vi "Test all Data Types in Variant.vi"() -> ()   [LabVIEW 2013]
uses:
  <vilib>/drjdpowell/Messenging/Core Messages/Message/MSG.lvclass
  <vilib>/drjdpowell/Messenging/Core Messages/Message/MSG.lvclass/MSG.ctl
  <vilib>/drjdpowell/Messenging/Core Messages/MSG Library/Write Message (dataless).vi
  <vilib>/drjdpowell/Messenging/Core Messages/MSG Library/Extract (no data).vi
  <vilib>/drjdpowell/Messenging/Core Messages/Message/Label Message.vi
  <vilib>/drjdpowell/Messenging/Core Messages/Message/Overwrite Reply Address.vi
  <vilib>/drjdpowell/Messenging/Core Messengers/Send/Send.lvclass
  JSONtext.lvlib
  <vilib>/drjdpowell/Messenging/Core Messages/MSG Library/SendMSG.lvlib
panel:
  out "x = y?":T1
  out "Occurence valid":bool
  out "error out":errorcluster
  out "Queue refun Valid":bool
  out "<JSON>":string
  out "subVariant":variant
  out "Label":string
  out "Variant out":variant
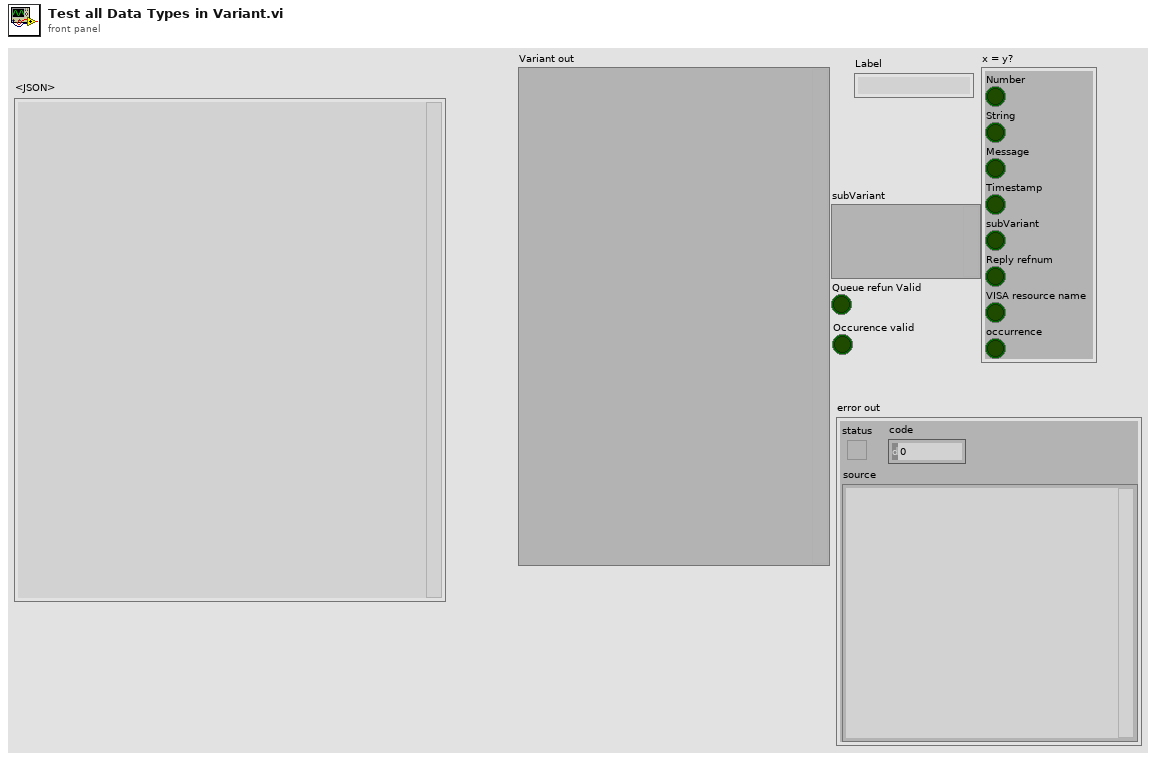
[diagram p1: front panel]
types:
  T1 = cluster{"Number":bool, "String":bool, "Message":bool, "Timestamp":bool, "subVariant":bool, "Reply refnum":bool, "VISA resource name":bool, "occurrence":bool}
  T2 = cluster{"Number":i32, "String":string, "Message":refnum<class "MSG.lvclass">, "Timestamp":timestamp, "subVariant":variant, "Reply refnum":refnum<queue>, "VISA resource name":refnum<visa-resource-name>, "occurrence":refnum<k4>}
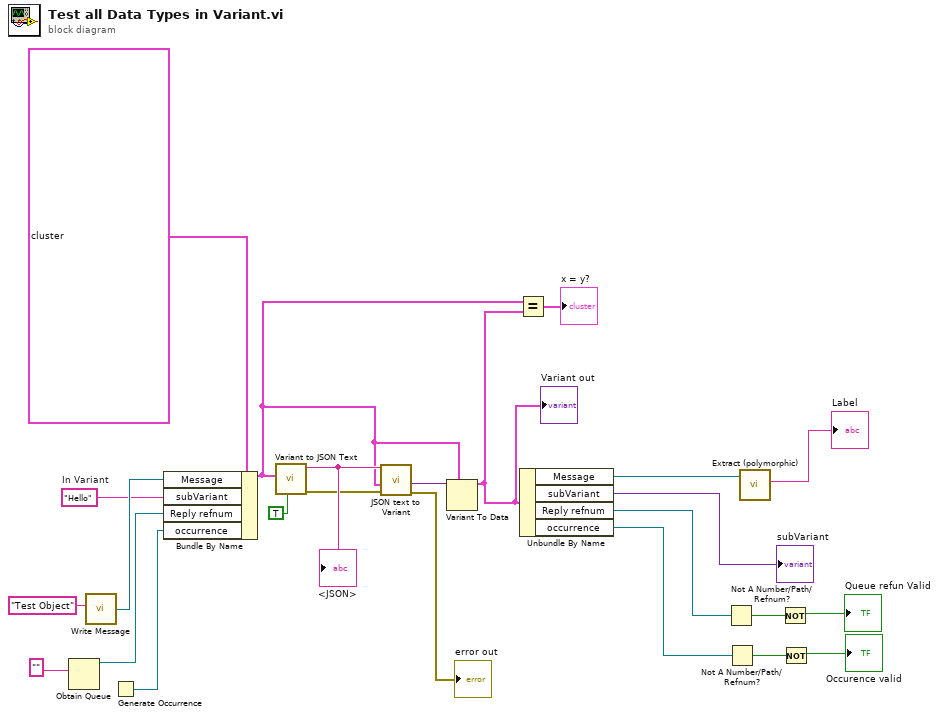
[diagram p0: block diagram]
diagram:
  w18 = "Hello"  # In Variant
  n1 = Obtain Queue(element data type="") -> (queue out=w14:refnum<queue>)  [unwired: 4 in, 2 out]
  n2 = call-poly <vilib>:"Write Message.vi"("Label"="Test Object") -> ("Message"=w22:refnum<class "MSG.lvclass">)  [unwired: 7 in]
  n3 = Generate Occurrence() -> (w7:refnum<k4>)
  n4 = Bundle By Name(cluster=T2 {"Number"=1234, "String"="Hello", "Message"=refnum, "Timestamp"=timestamp(3557316526.864 s since 1904-01-01), "subVariant"=variant, "Reply refnum"=refnum, "VISA resource name"="COM3", "occurrence"=refnum}, "Message"=w22, "subVariant"=w18, "Reply refnum"=w14, "occurrence"=w7) -> (w2:T2)
  n5 = call "Variant to JSON Text.vi"("Pretty Print?"=TRUE, "Variant"=w2) -> ("error out"=w8:errorcluster, "<JSON>"=w24:string)  [unwired: 8 in]
  "<JSON>" <- w24
  n6 = call "JSON text to Variant.vi"("error in (no error)"=w8, "Variant (Data Type)"=w2, "JSON"=w24) -> ("error out"=→"error out":errorcluster, "Variant out"=w21:variant)  [unwired: 7 in]
  n7 = Variant To Data(type=w2, Variant=w21) -> (data=w3:T2)  [unwired: 1 in, 1 out]
  "Variant out" <- w3
  n8 = Equal?(x=w2, y=w3) -> (x = y?=→"x = y?":T1)
  n9 = Unbundle By Name(w3) -> ("Message"=w20:refnum<class "MSG.lvclass">, "subVariant"=→"subVariant":variant, "Reply refnum"=w12:refnum<queue>, "occurrence"=w4:refnum<k4>)
  n10 = Not A Number/Path/Refnum?(number/path/refnum=w12) -> (NaN/Path/Refnum?=w11:bool)
  n11 = Not A Number/Path/Refnum?(number/path/refnum=w4) -> (NaN/Path/Refnum?=w5:bool)
  n12 = call-poly <vilib>:"Extract (polymorphic).vi"("Message"=w20) -> ("Label"=→"Label":string)  [unwired: 8 in, 2 out]
  n13 = Not(x=w11) -> (.not. x?=→"Queue refun Valid":bool)
  n14 = Not(x=w5) -> (.not. x?=→"Occurence valid":bool)
